vi "intersect_rays.vi"(5 "dt":dbl, 7 "t0":timestamp, 8 "Sensor 2 directions":T2, 9 "Sensor 2 base":dbl[](array[numeric]), 10 "Sensor 1 directions":T2, 11 "Sensor 1 base":dbl[](array[numeric])) -> (0 "Match error":waveform(dbl), 2 "XYZ":T1)   [LabVIEW 2010]
uses:
  <vilib>/Analysis/Matrix/Datatypes/RealMatrix.ctl
  <vilib>/Analysis/baseanly.llb/Real Dot Product.vi
  utilities/labview/magnitude_single.vi
  <vilib>/Analysis/NI_AALBase.lvlib
  <vilib>/Analysis/Matrix/NI_Matrix.lvlib
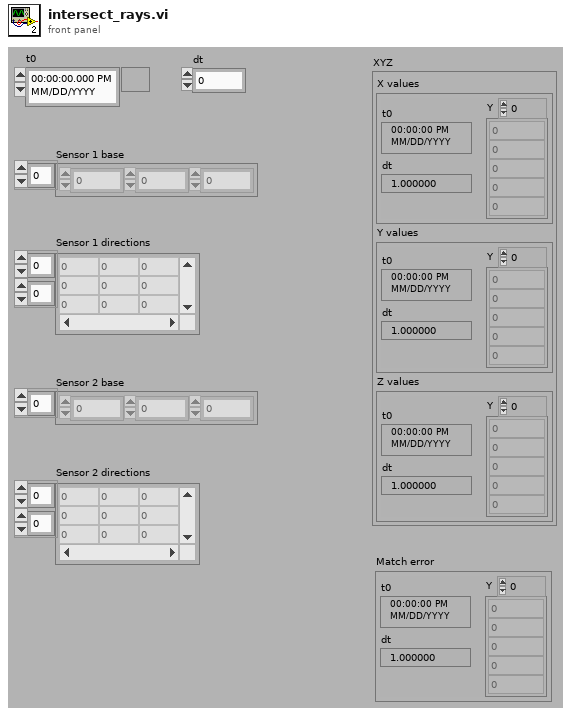
[diagram p1: front panel]
types:
  T1 = cluster{"X values":waveform(dbl), "Y values":waveform(dbl), "Z values":waveform(dbl)}
  T2 = typedef "NI_Matrix.lvlib/RealMatrix.ctl" = dbl[][]
  T3 = cluster{waveform(dbl), waveform(dbl), waveform(dbl)}
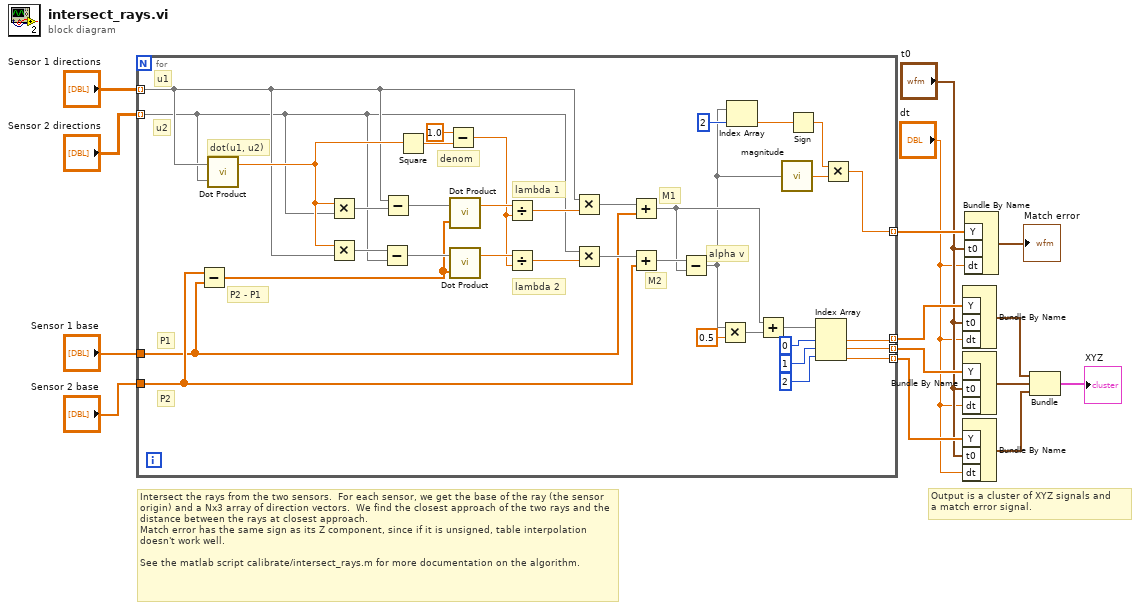
[diagram p0: block diagram]
diagram:
  # "Output is a cluster of XYZ signals and \na match error signal."
  # "Intersect the rays from the two sensors.  For each sensor, we get the base of the ray (the sensor origin) and a Nx3 array of direction vectors.  We find the closest approach of the two rays and the distance between the rays at closest approach. \nMatch error has the same sign as its Z component, since if it is unsigned, table interpolation doesn't work well.  \n\nSee the matlab script calibrate/intersect_rays.m for more documentation on the algorithm."
  n1 = for {
    tunnel: "Sensor 1 directions" -> [w41] mode=indexing
    tunnel: "Sensor 1 base" -> [w32]
    tunnel: "Sensor 2 base" -> [w35]
    tunnel: "Sensor 2 directions" -> [w39] mode=indexing
    tunnel: [w27] -> w6 mode=indexing
    tunnel: [w26] -> w5 mode=indexing
    tunnel: [w25] -> w4 mode=indexing
    tunnel: [w17] -> w3 mode=indexing
    # "alpha v"
    # "M2"
    # "M1"
    # "lambda 2"
    # "lambda 1"
    # "P2"
    # "P1"
    # "u1"
    # "u2"
    # "denom"
    # "P2 - P1"
    # "dot(u1, u2)"
    n2 = Subtract ("Subtract.vi")(x=w35, y=w32) -> (x-y=w24:dbl[])
    n3 = call-poly <vilib>:"Dot Product.vi"("Y Vector"=w39, "X Vector"=w41) -> ("X * Y"=w49:dbl)  [unwired: 1 out]
    n4 = Multiply(x=w49, y=w39) -> (x*y=w47:dbl[])
    n5 = Multiply(x=w49, y=w41) -> (x*y=w48:dbl[])
    n6 = Subtract(x=w48, y=w39) -> (x-y=w45:dbl[])
    n7 = Subtract(x=w41, y=w47) -> (x-y=w46:dbl[])
    n8 = Square(x=w49) -> (x^2=w51:dbl)
    n9 = Subtract(x=1.0, y=w51) -> (x-y=w42:dbl)
    n10 = call-poly <vilib>:"Dot Product.vi"("Y Vector"=w24, "X Vector"=w46) -> ("X * Y"=w44:dbl)  [unwired: 1 out]
    n11 = call-poly <vilib>:"Dot Product.vi"("Y Vector"=w24, "X Vector"=w45) -> ("X * Y"=w43:dbl)  [unwired: 1 out]
    n12 = Divide(x=w44, y=w42) -> (x/y=w40:dbl)
    n13 = Divide(x=w43, y=w42) -> (x/y=w38:dbl)
    n14 = Multiply(x=w41, y=w40) -> (x*y=w37:dbl[])
    n15 = Multiply(x=w39, y=w38) -> (x*y=w36:dbl[])
    n16 = Add(x=w37, y=w32) -> (x+y=w22:dbl[])
    n17 = Add(x=w36, y=w35) -> (x+y=w34:dbl[])
    n18 = Subtract(x=w34, y=w22) -> (x-y=w16:dbl[])
    n19 = Multiply(x=w16, y=0.5) -> (x*y=w23:dbl[])
    n20 = Index Array(array=w16, index=2) -> (element=w20:dbl)
    n21 = Add(x=w22, y=w23) -> (x+y=w31:dbl[])
    n22 = call-poly "magnitude.vi"("vector"=w16) -> ("vector magnitude"=w19:sgl)  [unwired: 4 in]
    n23 = Sign(1:w20) -> (0:w18:dbl)
    n24 = Index Array(array=w31, index #1=0 ("index"), index #2=1 ("index"), index #3=2 ("index")) -> (element #1=w27:dbl, element #2=w26:dbl, element #3=w25:dbl)
    n25 = Multiply(x=w18, y=w19) -> (x*y=w17:dbl)
  }
  n26 = Bundle By Name("Y"=w6, "t0"="t0", "dt"="dt") -> (w11:waveform(dbl))  [unwired: 1 out]
  n27 = Bundle By Name("Y"=w5, "t0"="t0", "dt"="dt") -> (w10:waveform(dbl))  [unwired: 1 out]
  n28 = Bundle By Name("Y"=w4, "t0"="t0", "dt"="dt") -> (w9:waveform(dbl))  [unwired: 1 out]
  n29 = Bundle By Name("Y"=w3, "t0"="t0", "dt"="dt") -> (→"Match error":waveform(dbl))  [unwired: 1 out]
  n30 = Bundle(w11, w10, w9) -> (→"XYZ":T3)  [unwired: 1 out]
